vi "dfd_Match Conj Pair Zeros and Poles.vi"(10 "conj poles":cdb[](array[numeric]), 11 "conj zeros":cdb[](array[numeric])) -> (1 "matched z&p":cluster{"zeros":cdb[], "poles":cdb[]}[](array[cluster]), 2 "remaining poles":cdb[](array[numeric]), 3 "remaining zeros":cdb[](array[numeric]))   [LabVIEW 2017, in "NI_DigFilterLicensed.lvlib"]
uses:
  <vilib>/addons/Digital Filter Design/NI_DigFilterLicensed.lvlib
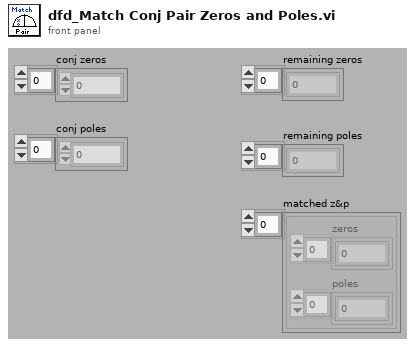
[diagram p1: front panel]
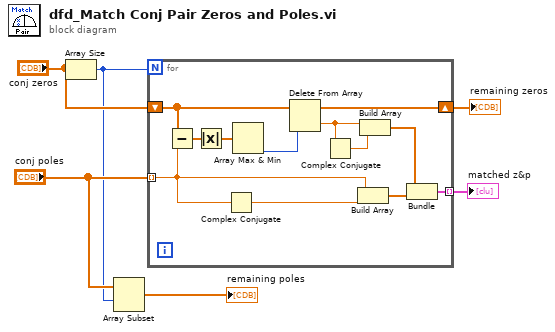
[diagram p0: block diagram]
diagram:
  n1 = Array Size(array="conj zeros") -> (size(s)=w2:i32)
  n2 = Array Subset(array="conj poles", index=w2) -> (→"remaining poles":cdb[])  [unwired: 1 in]
  n3 = for {
    N: w2 -> [_]
    shift-right: [w15] -> w4
    shift-left: "conj zeros" -> [w18]
    tunnel: [w7] -> w5 mode=indexing
    tunnel: "conj poles" -> [w10] mode=indexing
    n4 = Subtract(x=w18, y=w10) -> (x-y=w17:cdb[])
    n5 = Absolute Value(x=w17) -> (abs(x)=w16:dbl[])
    n6 = Complex Conjugate(1:w10) -> (0:w11:cdb)
    n7 = Array Max & Min(array=w16) -> (min index (indices)=w14:i32)  [unwired: 3 out]
    n8 = Delete From Array(array=w18, index=w14) -> (deleted portion=w12:cdb, array with subset deleted=w15:cdb[])  [unwired: 1 in]
    n9 = Complex Conjugate(1:w12) -> (0:w13:cdb)
    n10 = Build Array(w10, w11) -> (w8:cdb[])
    n11 = Build Array(w12, w13) -> (w9:cdb[])
    n12 = Bundle(w9, w8) -> (w7:cluster{cdb[], cdb[]})  [unwired: 1 out]
  }
  "remaining zeros" <- w4
  "matched z&p" <- w5
